vi "Log Errors.vi"(7 "section identifier":string, 10 "errors in":errorcluster[](array[cluster]), 11 "log file":path=path "c:/ni-rt/VeriStand/Custom Devices/Errors.txt") -> ()   [LabVIEW 2020]
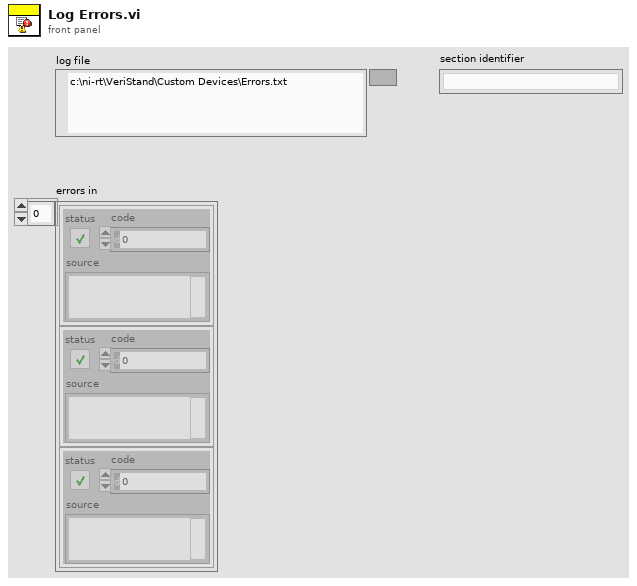
[diagram p1: front panel]
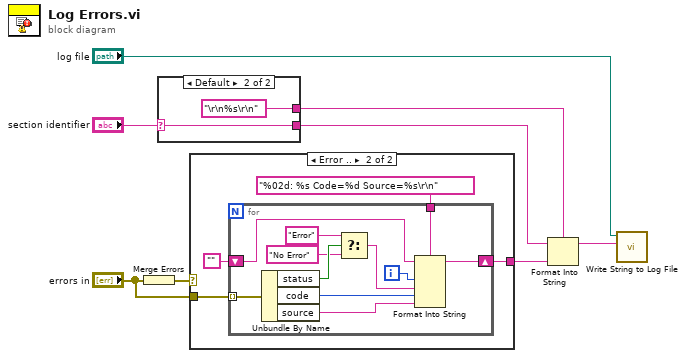
[diagram p0: block diagram]
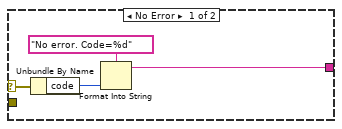
[diagram p2: hidden frame]
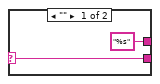
[diagram p3: hidden frame]
diagram:
  n1 = Merge Errors("errors in") -> (w7:errorcluster)
  n2 = case shown="Default" "section identifier" {
    selector: "section identifier" -> [w10 w11]
    tunnel: ["%s" ("format string") "\r\n%s\r\n" ("format string")] -> w5
    tunnel: [w10 w11] -> w1
    frame "" {
    }
    frame Default {
    }
  }
  n3 = case shown="Error .." w7 {
    selector: w7 -> [w16 _]
    tunnel: [w13 w19] -> w6
    tunnel: "errors in" -> [_ w20]
    frame No Error {
      n4 = Unbundle By Name(w16) -> ("code"=w15:i32)
      n5 = Format Into String(format string="No error. Code=%d", w15) -> (resulting string=w13:string)  [unwired: 2 in, 1 out]
    }
    frame Error {
      n6 = for {
        tunnel: w20 -> [w31] mode=indexing
        shift-right: [w23] -> w19
        shift-left: "" -> [w22]
        tunnel: "%02d: %s Code=%d Source=%s\r\n" ("format string") -> [w21]
        i -> [w24]
        n7 = Unbundle By Name(w31) -> ("status"=w30:bool, "code"=w26:i32, "source"=w25:string)
        n8 = Select(t="Error" ("source"), s=w30, f="No Error" ("source")) -> (s? t:f=w27:string)
        n9 = Format Into String(format string=w21, initial string=w22, w24, w27, w26, w25) -> (resulting string=w23:string)  [unwired: 1 in, 1 out]
      }
    }
  }
  n10 = Format Into String(format string=w5, initial string=w1, w6) -> (resulting string=w4:string)  [unwired: 1 in, 1 out]
  n11 = call "Write String to Log File.vi"("string to log"=w4, "log file"="log file") -> ()  [unwired: 9 in, 1 out]
